vi "_GetSockOpt.vi"(0 "Socket":u32, 3 "OptionName":i32, 7 "I32 mode? (T)":bool=TRUE, 11 "Error In":errorcluster, 12 "Level":i32) -> (4 "Socket Out":u32 format="%x", 6 "Value (I32)":i32, 8 "Mode Out":bool=TRUE, 10 "Value":u8[](array[numeric]), 15 "Error Out":errorcluster)   [LabVIEW 2018]
uses:
  ws2_32.dll
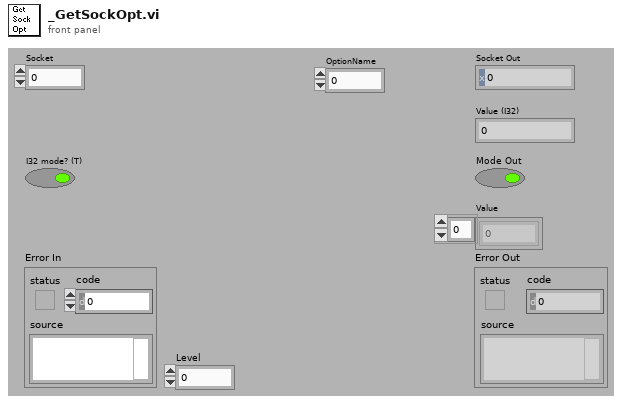
[diagram p1: front panel]
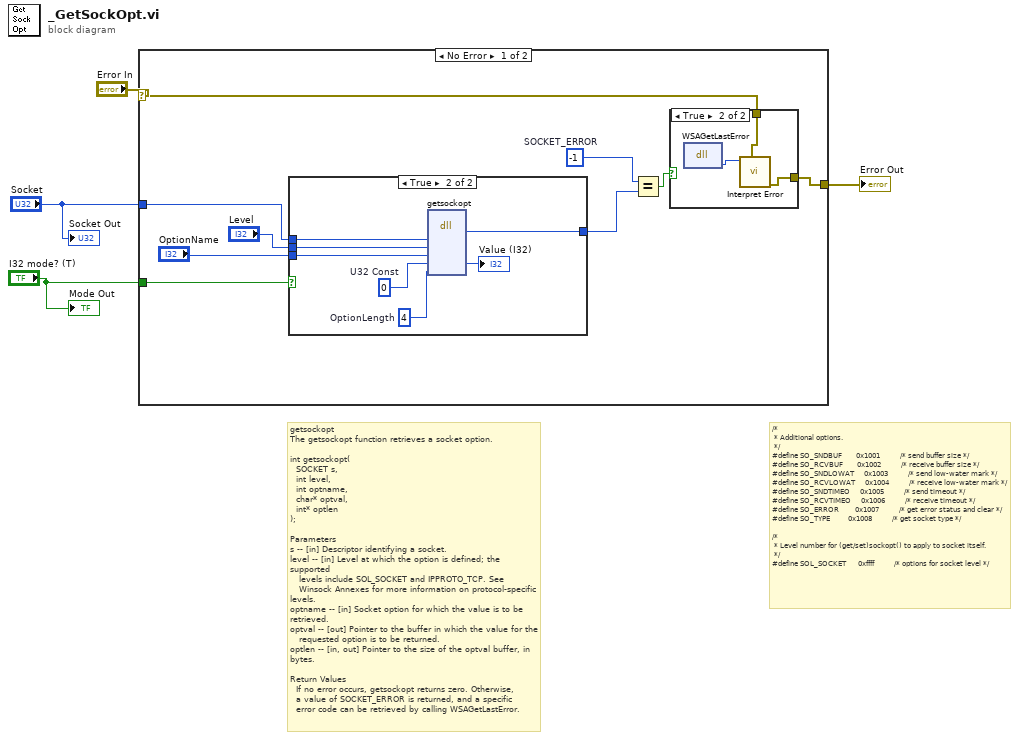
[diagram p0: block diagram]
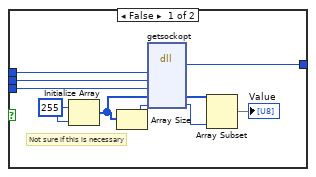
[diagram p2: hidden frame]
diagram:
  # "/*\n * Additional options.\n */\n#define SO_SNDBUF       0x1001          /* send buffer size */\n#define SO_RCVBUF       0x1002          /* receive buffer size */\n#define SO_SNDLOWAT     0x1003          /* send low-water mark */\n#define SO_RCVLOWAT     0x1004          /* receive low-water mark */\n#define SO_SNDTIMEO     0x1005          /* send timeout */\n#define SO_RCVTIMEO     0x1006          /* receive timeout */\n#define SO_ERROR        0x1007          /* get error status and clear */\n#define SO_TYPE         0x1008          /* get socket type */\n\n/*\n * Level number for (get/set)sockopt() to apply to socket itself.\n */\n#define SOL_SOCKET      0xffff          /* options for socket level */"
  # "getsockopt\nThe getsockopt function retrieves a socket option.\n\nint getsockopt(\n  SOCKET s,\n  int level,\n  int optname,\n  char* optval,\n  int* optlen\n);\n\nParameters\ns -- [in] Descriptor identifying a socket. \nlevel -- [in] Level at which the option is defined; the supported \n   levels include SOL_SOCKET and IPPROTO_TCP. See \n   Winsock Annexes for more information on protocol-specific levels. \noptname -- [in] Socket option for which the value is to be retrieved. \noptval -- [out] Pointer to the buffer in which the value for the \n   requested option is to be returned. \noptlen -- [in, out] Pointer to the size of the optval buffer, in bytes. \n\nReturn Values\n  If no error occurs, getsockopt returns zero. Otherwise, \n  a value of SOCKET_ERROR is returned, and a specific\n  error code can be retrieved by calling WSAGetLastError."
  n1 = case shown="No Error" "Error In" {
    selector: "Error In" -> [w12 w35]
    tunnel: [w11 w35] -> w3
    tunnel: "Socket" -> [w6 _]
    tunnel: "I32 mode? (T)" -> [w5 _]
    frame No Error {
      w13 = -1  # SOCKET_ERROR
      n2 = case shown="True" w5 {
        tunnel: [w23 w30] -> w10
        tunnel: "OptionName" -> [w22 w29]
        tunnel: "Level" -> [w21 w28]
        tunnel: w6 -> [w20 w27]
        frame False {
          w19 = u8 255
          # "Not sure if this is necessary"
          n3 = Initialize Array(w19, w19) -> (w17:u8[])
          n4 = Array Size(array=w17) -> (size(s)=w18:i32)
          n5 = dll-call lib="ws2_32.dll" fn="getsockopt" label="GetSockOpt"("Socket"=w20, "Level"=w21, "OptionName"=w22, "OptionValue"=w17, "OptionLength"=w18) -> (w23:i32, "OptionValue"=w14:u8[], "OptionLength"=w15:i32)  [unwired: 6 in, 2 out]
          n6 = Array Subset(array=w14, length=w15) -> (→"Value":u8[])  [unwired: 1 in]
        }
        frame True {
          w24 = 4  # OptionLength
          w25 = u32 0  # U32 Const
          n7 = dll-call lib="ws2_32.dll" fn="getsockopt" label="GetSockOpt"("Socket"=w27, "Level"=w28, "OptionName"=w29, "OptionValue"=w25, "OptionLength"=w24) -> (w30:i32, "OptionValue"=→"Value (I32)":i32)  [unwired: 7 in, 2 out]
        }
      }
      n8 = Equal?(x=w13, y=w10) -> (x = y?=w9:bool)
      n9 = case shown="True" w9 {
        tunnel: w12 -> [w31 w33]
        tunnel: [w31 w32] -> w11
        frame False {
        }
        frame True {
          n10 = dll-call lib="ws2_32.dll" fn="WSAGetLastError"() -> (w34:i32)  [unwired: 3 in, 2 out]
          n11 = call "Interpret Error.vi"("Error In"=w33, "Code"=w34) -> ("Error Out"=w32:errorcluster)  [unwired: 9 in]
        }
      }
    }
    frame Error {
    }
  }
  "Error Out" <- w3
  "Socket Out" <- "Socket"
  "Mode Out" <- "I32 mode? (T)"
